vi "Destroy.vi"(8 "error in (no error)":errorcluster, 11 "Executioner in":refnum<class "Executioner.lvclass">) -> (0 "error out":errorcluster)   [LabVIEW 2019, in "Test Executive.lvlib" / "Executioner.lvclass"]
uses:
  <vilib>/gpm_packages/@cs/test-executive/Source/Test Executive/Executioner/Executioner.lvclass
  <vilib>/gpm_packages/@cs/test-executive/Source/Test Executive/Executioner/Executioner.lvclass/Executioner.ctl
  <vilib>/gpm_packages/@cs/lookup-table/Source/LookupTable/LookupTable.lvclass
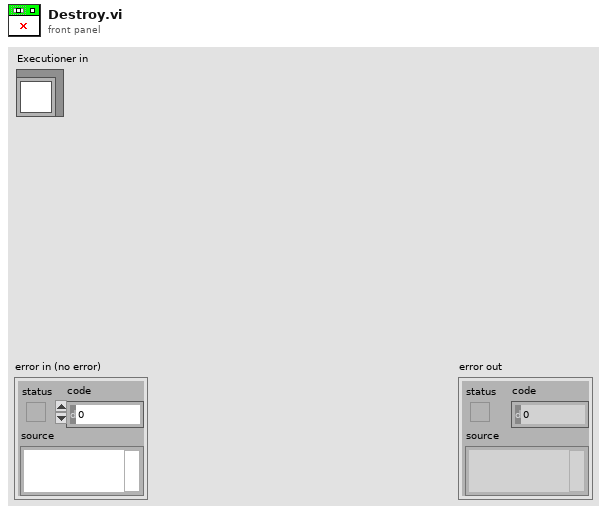
[diagram p1: front panel]
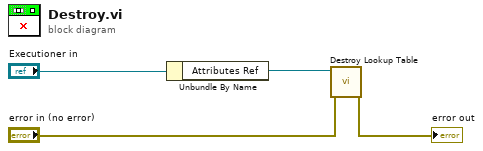
[diagram p0: block diagram]
diagram:
  n1 = Unbundle By Name("Executioner in") -> ("Attributes Ref"=w3:refnum<data-value>)
  n2 = call <vilib>:"Destroy Lookup Table.vi"("error in (no error)"="error in (no error)", "LookupTable Reference"=w3) -> ("error out"=→"error out":errorcluster)  [unwired: 9 in]
